vi "Untitled 1.vi"() -> ()   [LabVIEW 2013]
panel:
  in  "Enter":bool
  in  "User Input":string
  in  "Right Buttons":T1
  out "Right Menu":T2
  in  "Left Buttons":T1
  out "Left Menu":T2
  in  "Card Simulator":bool
  out "ATM Messages":string
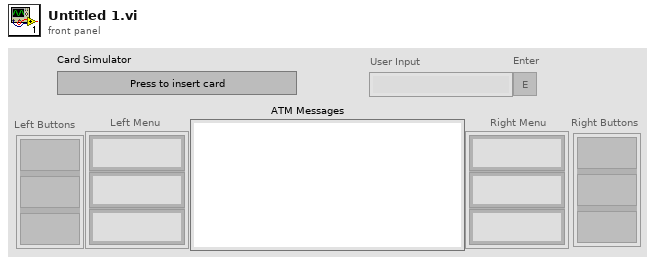
[diagram p1: front panel]
types:
  T1 = cluster{"Func Button":bool, "Func Button 2":bool, "Func Button 3":bool}
  T2 = cluster{"RFS String":string, "RFS String 2":string, "RFS String 3":string}
  T3 = cluster{"Right Buttons":refnum<vi>, "Left Buttons":refnum<vi>, "Left Menu":refnum<vi>, "Right Menu":refnum<vi>, "User Input":refnum<vi>, "Card Simulator":refnum<vi>}
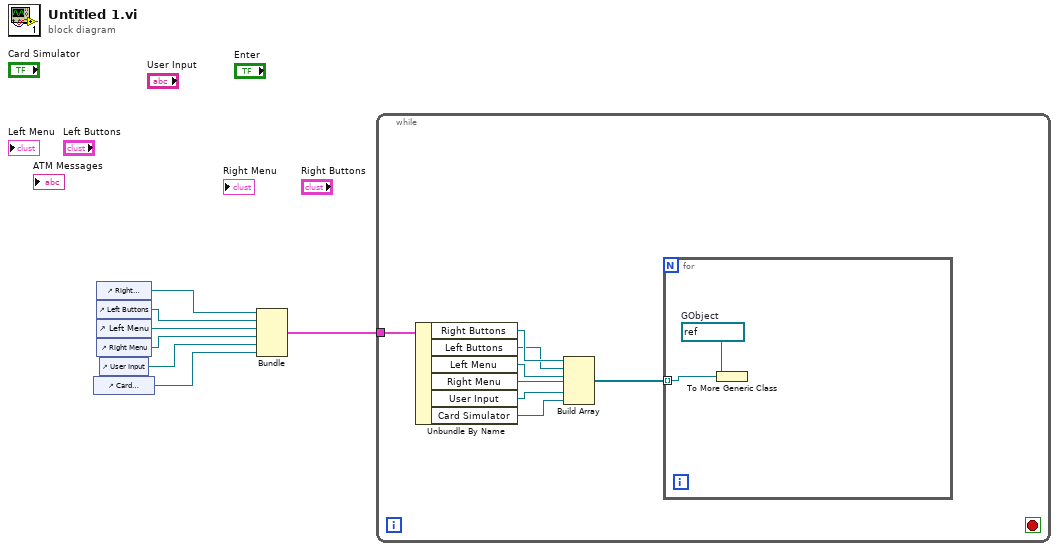
[diagram p0: block diagram]
diagram:
  n1 = control-ref of="Card Simulator"() -> (w2:refnum<vi>)
  n2 = control-ref of="Right Buttons"() -> (w7:refnum<vi>)
  n3 = control-ref of="Left Buttons"() -> (w6:refnum<vi>)
  n4 = control-ref of="Left Menu"() -> (w5:refnum<vi>)
  n5 = control-ref of="Right Menu"() -> (w4:refnum<vi>)
  n6 = control-ref of="User Input"() -> (w3:refnum<vi>)
  n7 = Bundle("Right Buttons"=w7, "Left Buttons"=w6, "Left Menu"=w5, "Right Menu"=w4, "User Input"=w3, "Card Simulator"=w2) -> (w1:T3)  [unwired: 1 in]
  n8 = while {
    tunnel: w1 -> [w15]
    stop <- _ stop-if-true
    n9 = Unbundle By Name(w15) -> ("Right Buttons"=w14:refnum<vi>, "Left Buttons"=w13:refnum<vi>, "Left Menu"=w12:refnum<vi>, "Right Menu"=w9:refnum<vi>, "User Input"=w11:refnum<vi>, "Card Simulator"=w10:refnum<vi>)
    n10 = Build Array(w14, w13, w12, w9, w11, w10) -> (w8:refnum<vi>[])
    n11 = for {
      tunnel: w8 -> [w17] mode=indexing
      w16 = refnum<vi> refnum  # GObject
      n12 = To More Generic Class(target class=w16, reference=w17) -> ()  [unwired: 1 out]
    }
  }
